vi "makeDecisions.vi"(8 "error in (no error)":errorcluster, 10 "model":refnum<class "Model.lvclass">, 11 "SamplingState in":refnum<class "SamplingState.lvclass">) -> (0 "error out":errorcluster, 2 "model 2":refnum<class "Model.lvclass">, 3 "SamplingState out":refnum<class "SamplingState.lvclass">)   [LabVIEW 2013, in "SamplingState.lvclass"]
uses:
  SamplingState.lvclass
  Model/Model/Model.lvclass
  LogBridgeDataState/LogBridgeDataState.lvclass
  Typedefs/StateSelector.ctl
  Typedefs/AITDTTypedefs.lvlib
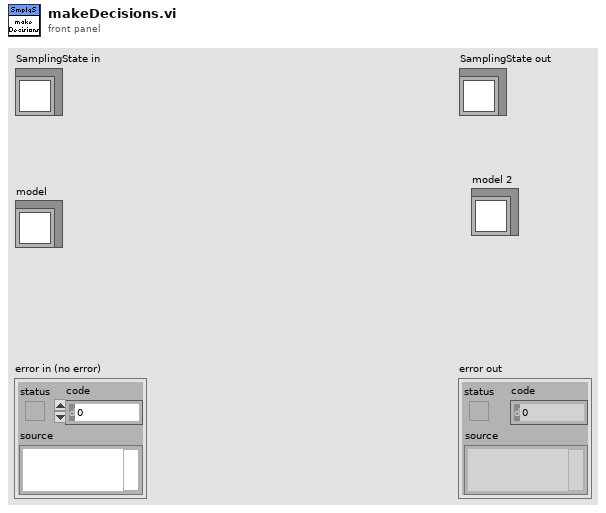
[diagram p1: front panel]
types:
  T1 = typedef "AITDTTypedefs.lvlib/StateSelector.ctl" = enum16{"AwaitingSetpointAcknowledgmentState", "EndingCycleState", "FaultState", "OffState", "PausingState", "RequestingNewSetpointState", "SamplingState", "SettlingState", "SoakingState", "StabilizingState", "StandbyState", "StoppedState", "TransitioningTemperatureState"}
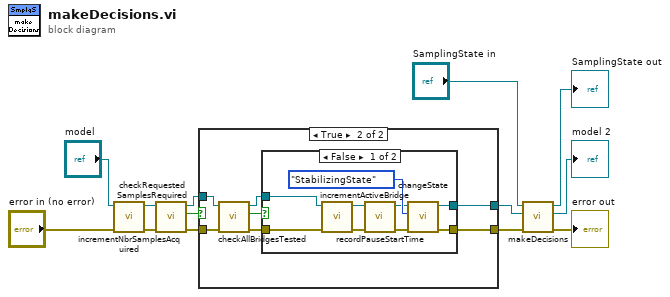
[diagram p0: block diagram]
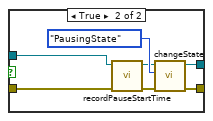
[diagram p3: hidden frame]
diagram:
  n1 = call "incrementNbrSamplesAcquired.vi"("error in (no error)"="error in (no error)", "Model in"="model") -> ("error out"=w1:errorcluster, "Model out"=w3:refnum<class "Model.lvclass">)  [unwired: 8 in]
  n2 = call "checkRequestedSamplesRequired.vi"("error in (no error)"=w1, "Model in"=w3) -> ("error out"=w5:errorcluster, "requestedSamplesAcquiredIsTrue==T"=w6:bool, "Model out"=w7:refnum<class "Model.lvclass">)  [unwired: 7 in]
  n3 = case shown="True" w6 {
    tunnel: [w14 w20] -> w9
    tunnel: w5 -> [w15 w18]
    tunnel: [w15 w17] -> w8
    tunnel: w7 -> [w14 w16]
    frame False {
    }
    frame True {
      n4 = call "checkAllBridgesTested.vi"("error in (no error)"=w18, "Model in"=w16) -> ("error out"=w19:errorcluster, "allBridgesTestedIsTrue"=w22:bool, "Model out"=w21:refnum<class "Model.lvclass">)  [unwired: 7 in]
      n5 = case shown="False" w22 {
        tunnel: w21 -> [w30 w35]
        tunnel: [w27 w37] -> w20
        tunnel: w19 -> [w29 w33]
        tunnel: [w28 w36] -> w17
        frame False {
          n6 = call "incrementActiveBridge.vi"("error in (no error)"=w29, "Model in"=w30) -> ("error out"=w25:errorcluster, "Model out"=w26:refnum<class "Model.lvclass">)  [unwired: 8 in]
          n7 = call "recordPauseStartTime.vi"("error in (no error)"=w25, "Model in"=w26) -> ("error out"=w24:errorcluster, "Model out"=w23:refnum<class "Model.lvclass">)  [unwired: 8 in]
          n8 = call "changeState.vi"("error in (no error)"=w24, "State:"=StateSelector."StabilizingState", "Model in"=w23) -> ("error out"=w28:errorcluster, "Model out"=w27:refnum<class "Model.lvclass">)  [unwired: 7 in]
        }
        frame True {
          n9 = call "recordPauseStartTime.vi"("error in (no error)"=w33, "Model in"=w35) -> ("error out"=w32:errorcluster, "Model out"=w34:refnum<class "Model.lvclass">)  [unwired: 8 in]
          n10 = call "changeState.vi"("error in (no error)"=w32, "State:"=StateSelector."PausingState", "Model in"=w34) -> ("error out"=w36:errorcluster, "Model out"=w37:refnum<class "Model.lvclass">)  [unwired: 7 in]
        }
      }
    }
  }
  n11 = call-parent "makeDecisions.vi"("error in (no error)"=w8, "model"=w9, "EnabledState in"="SamplingState in") -> ("error out"=→"error out":errorcluster, "model 2"=→"model 2":refnum<class "Model.lvclass">, "EnabledState out"=→"SamplingState out":refnum<class "SamplingState.lvclass">)  [unwired: 6 in]
